vi "NILIA_LPF_Settings.vi"(9 "rolloff":T1(ring), 10 "TC [sec]":dbl=0.25 format="%.2f", 11 "fs":dbl format="%.2f") -> (0 "3rd stages":i32, 1 "3rd decimation":i32, 2 "2nd stages":i32, 3 "2nd decimation":i32, 4 "settling time [sec]":dbl format="%.2f", 5 "1st stages":i32, 6 "actual TC [sec]":dbl format="%.2f", 7 "1st decimation":i32)   [LabVIEW 2009]
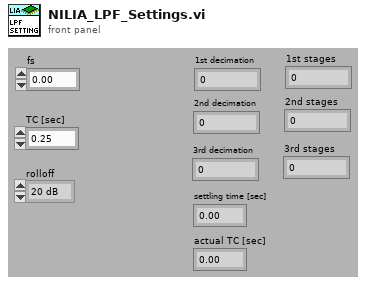
[diagram p1: front panel]
types:
  T1 = enum16{"20 dB", "40 dB", "60 dB", "80 dB", "100 dB", "120 dB", "140 dB", "160 dB", "180 dB", "200 dB"}
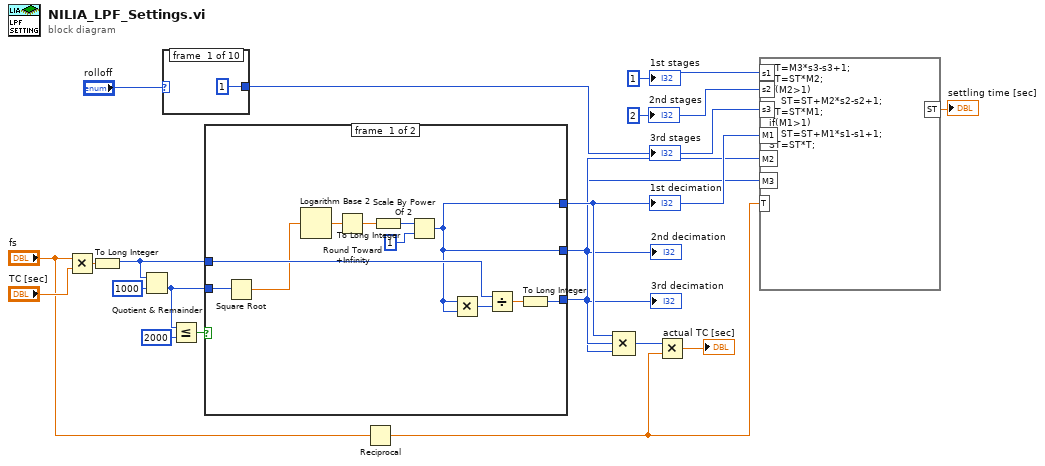
[diagram p0: block diagram]
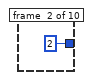
[diagram p2: hidden frame]
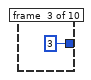
[diagram p3: hidden frame]
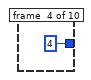
[diagram p4: hidden frame]
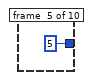
[diagram p5: hidden frame]
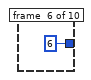
[diagram p6: hidden frame]
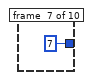
[diagram p7: hidden frame]
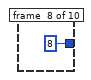
[diagram p8: hidden frame]
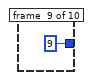
[diagram p9: hidden frame]
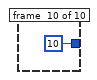
[diagram p10: hidden frame]
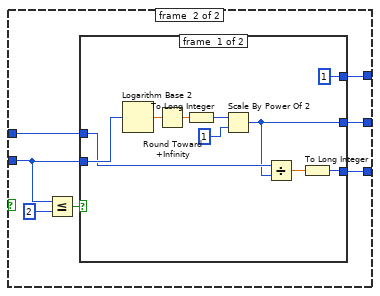
[diagram p11: hidden frame]
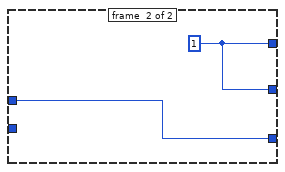
[diagram p12: hidden frame]
diagram:
  w11 = 2 ("2nd stages")
  w4 = 1 ("1st stages")
  n1 = Multiply(x="fs", y="TC [sec]") -> (x*y=w13:dbl)
  n2 = To Long Integer(number=w13) -> (32bit integer=w12:i32)
  n3 = Quotient & Remainder(x=w12, y=1000) -> (floor(x/y)=w16:i32)  [unwired: 1 out]
  n4 = case shown="\"200 dB\"" "rolloff" {
    tunnel: [1 2 3 4 5 6 7 8 9 10] -> w1
    frame #0 {
    }
    frame #1 {
    }
    frame #2 {
    }
    frame #3 {
    }
    frame #4 {
    }
    frame #5 {
    }
    frame #6 {
    }
    frame #7 {
    }
    frame #8 {
    }
    frame #9 {
    }
  }
  "3rd stages" <- w1
  n5 = Less Or Equal?(x=w16, y=2000) -> (x <= y?=w17:bool)
  n6 = case shown="False" w17 {
    tunnel: w12 -> [w39 w44]
    tunnel: w16 -> [w40 w41]
    tunnel: [w32 w43] -> w15
    tunnel: [w32 w42] -> w10
    tunnel: [w36 w45] -> w9
    frame #0 {
      n7 = Square Root(x=w40) -> (sqrt(x)=w31:dbl)
      n8 = Logarithm Base 2(1:w31) -> (0:w35:dbl)
      n9 = Round Toward +Infinity(x=w35) -> (ceil(x): smallest int >= x=w30:dbl)
      n10 = To Long Integer(number=w30) -> (32bit integer=w33:i32)
      n11 = Scale By Power Of 2(n=w33, x=1) -> (x*2^n=w32:i32)
      n12 = Multiply(x=w32, y=w32) -> (x*y=w38:i32)
      n13 = Divide(x=w39, y=w38) -> (x/y=w37:dbl)
      n14 = To Long Integer(number=w37) -> (32bit integer=w36:i32)
    }
    frame #1 {
      n15 = Less Or Equal?(x=w41, y=2) -> (x <= y?=w47:bool)
      n16 = case shown="False" w47 {
        tunnel: [w55 w58] -> w45
        tunnel: w44 -> [w52 w58]
        tunnel: [1 w59] -> w43
        tunnel: [w49 w59] -> w42
        tunnel: w41 -> [w53 _]
        frame #0 {
          n17 = Logarithm Base 2(1:w53) -> (0:w54:dbl)
          n18 = Round Toward +Infinity(x=w54) -> (ceil(x): smallest int >= x=w48:dbl)
          n19 = To Long Integer(number=w48) -> (32bit integer=w50:i32)
          n20 = Scale By Power Of 2(n=w50, x=1) -> (x*2^n=w49:i32)
          n21 = Divide(x=w52, y=w49) -> (x/y=w56:dbl)
          n22 = To Long Integer(number=w56) -> (32bit integer=w55:i32)
        }
        frame #1 {
          w59 = 1
        }
      }
    }
  }
  "1st decimation" <- w15
  "2nd decimation" <- w10
  "3rd decimation" <- w9
  n23 = Reciprocal(x="fs") -> (1/x=w5:dbl)
  n24 = Compound Arithmetic op=MULTIPLY(w15, w10, w9) -> (w8:i32)
  n25 = Multiply(x=w8, y=w5) -> (x*y=→"actual TC [sec]":dbl)
  n26 = formula code="ST=M3*s3-s3+1;\nST=ST*M2;\nif(M2>1)\n    ST=ST+M2*s2-s2+1;\nST=ST*M1;\nif(M1>1)\n    ST=ST+M1*s1-s1+1;\nST=ST*T;"("s1"=w4, "s2"=w11, "s3"=w1, "M1"=w15, "M2"=w10, "M3"=w9, "T"=w5) -> ("ST"=→"settling time [sec]":dbl)
  "2nd stages" <- w11
  "1st stages" <- w4
